vi "Find Curriculum.vi"(8 "error in (no error)":errorcluster, 10 "Array ot connected evices":string[](array[string]), 11 "Location of Examples":path) -> (0 "error out":errorcluster, 2 "Is the required hardware detected?":bool[](array[boolean]), 3 "Example File Paths":path[](array[path]))   [LabVIEW 2020]
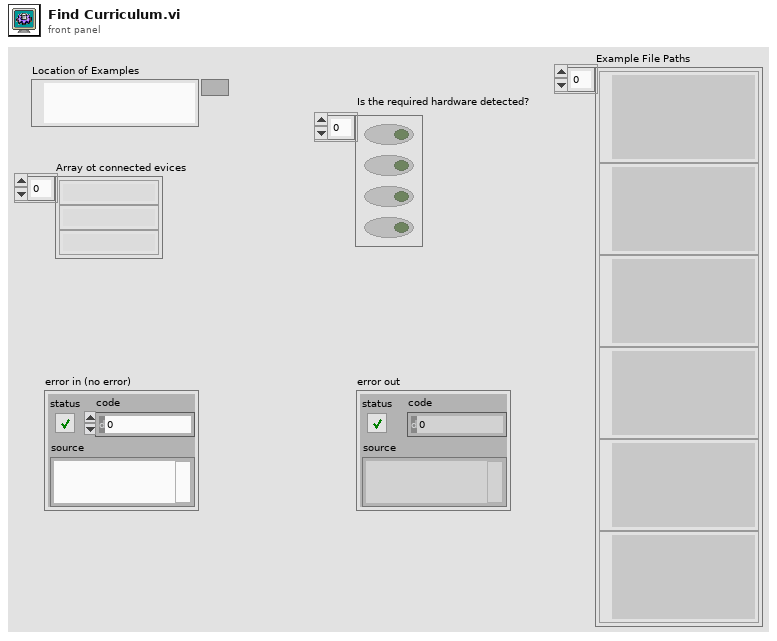
[diagram p1: front panel]
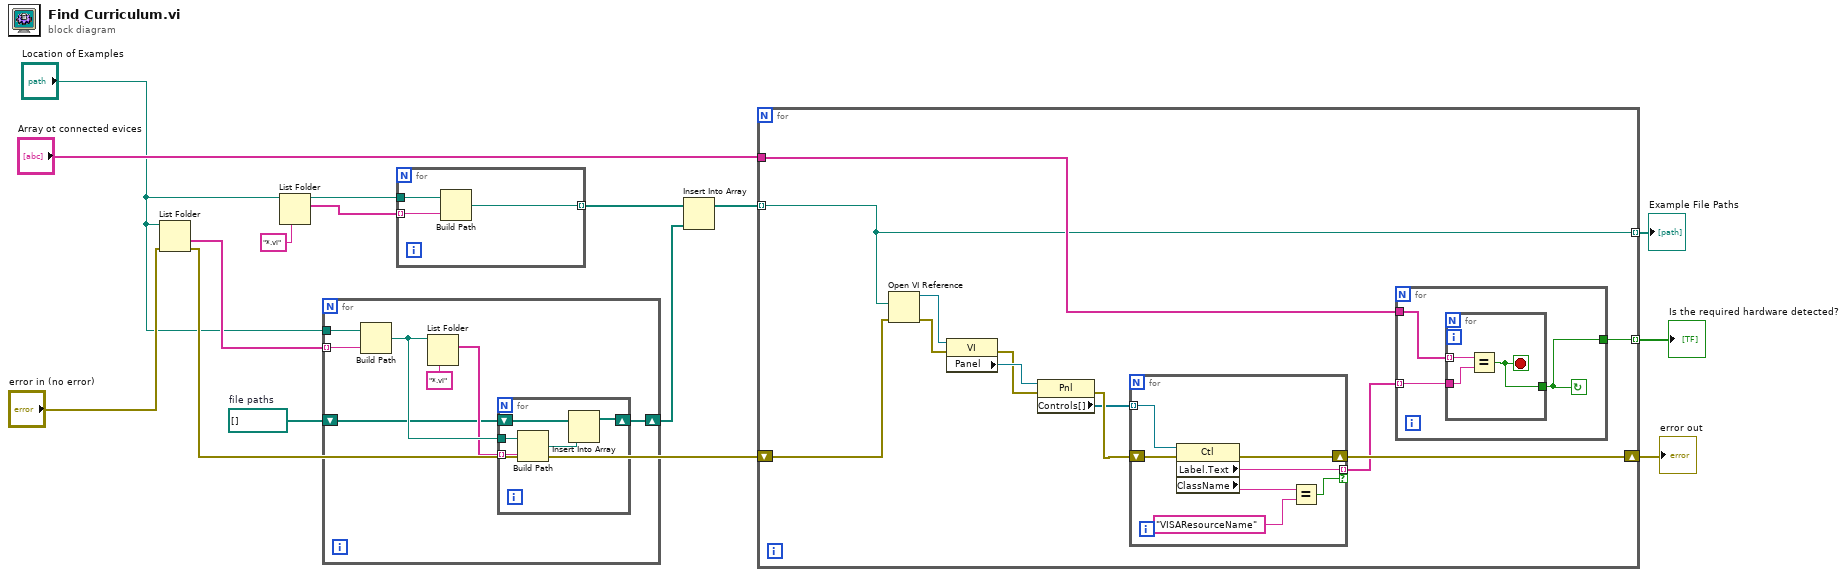
[diagram p0: block diagram]
diagram:
  w8 = path[] []  # file paths
  n1 = List Folder(path="Location of Examples", error in="error in (no error)") -> (folder names=w9:string[], error out=w11:errorcluster)  [unwired: 2 in, 2 out]
  n2 = List Folder(path="Location of Examples", pattern="*.vi") -> (path out=w4:path, filenames=w5:string[])  [unwired: 2 in, 2 out]
  n3 = for {
    tunnel: w9 -> [w22] mode=indexing
    tunnel: "Location of Examples" -> [w21]
    shift-right: [w17] -> w2
    shift-left: w8 -> [w16]
    n4 = Build Path(base path=w21, name or relative path=w22) -> (appended path=w19:path)
    n5 = List Folder(path=w19, pattern="*.vi") -> (filenames=w18:string[])  [unwired: 2 in, 3 out]
    n6 = for {
      tunnel: w19 -> [w27]
      tunnel: w18 -> [w26] mode=indexing
      shift-right: [w24] -> w17
      shift-left: w16 -> [w23]
      n7 = Build Path(base path=w27, name or relative path=w26) -> (appended path=w25:path)
      n8 = Insert Into Array(array=w23, new element=w25) -> (w24:path[])  [unwired: 1 in]
    }
  }
  n9 = for {
    tunnel: w5 -> [w29] mode=indexing
    tunnel: w4 -> [w30]
    tunnel: [w28] -> w3 mode=indexing
    n10 = Build Path(base path=w30, name or relative path=w29) -> (appended path=w28:path)
  }
  n11 = Insert Into Array(array=w3, new element=w2) -> (w1:path[])  [unwired: 1 in]
  n12 = for {
    tunnel: [w40] -> w13 mode=indexing
    tunnel: "Array ot connected evices" -> [w39]
    shift-right: [w35] -> w15
    shift-left: w11 -> [w38]
    tunnel: [w31] -> w10 mode=indexing
    tunnel: w1 -> [w31] mode=indexing
    n13 = Open VI Reference(vi path=w31, error in (no error)=w38) -> (vi reference=w42:refnum<vi>, error out=w37:errorcluster)  [unwired: 4 in]
    n14 = property class="VI"(reference=w42, error in=w37) -> (error out=w36:errorcluster, "Panel"=w41:refnum<vi>)  [unwired: 1 out]
    n15 = property class="Pnl"(reference=w41, error in=w36) -> (error out=w33:errorcluster, "Controls[]"=w32:refnum<vi>[])  [unwired: 1 out]
    n16 = for {
      tunnel: w32 -> [w55] mode=indexing
      tunnel: [w52] -> w34 mode=indexing if=w51
      shift-right: [w49] -> w35
      shift-left: w33 -> [w50]
      n17 = property class="Ctl"(reference=w55, error in=w50) -> (error out=w49:errorcluster, "Label.Text"=w52:string, "ClassName"=w54:string)  [unwired: 1 out]
      n18 = Equal?(x=w54, y="VISAResourceName") -> (x = y?=w51:bool)
    }
    n19 = for {
      tunnel: w34 -> [w45] mode=indexing
      tunnel: w39 -> [w44]
      tunnel: [w43] -> w40
      stop <- w43 continue-if-true
      n20 = for {
        tunnel: w45 -> [w47]
        tunnel: w44 -> [w48] mode=indexing
        tunnel: [w46] -> w43
        stop <- w46 stop-if-true
        n21 = Equal?(x=w48, y=w47) -> (x = y?=w46:bool)
      }
    }
  }
  "error out" <- w15
  "Is the required hardware detected?" <- w13
  "Example File Paths" <- w10
